vi "fpga_Fund Filter Constant.vi"() -> (0 "Total Delay":u8=24, 1 "Start":fxp<+/-,4,4>=1.0, 2 "LP2 delay":u8, 3 "LP1 delay":u8=2)   [LabVIEW 2012, in "NI_EP_Protection_FPGA.lvlib"]
uses:
  <vilib>/addons/Electrical Power/Protection/NI_EP_Protection_FPGA.lvlib
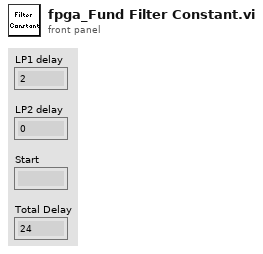
[diagram p1: front panel]
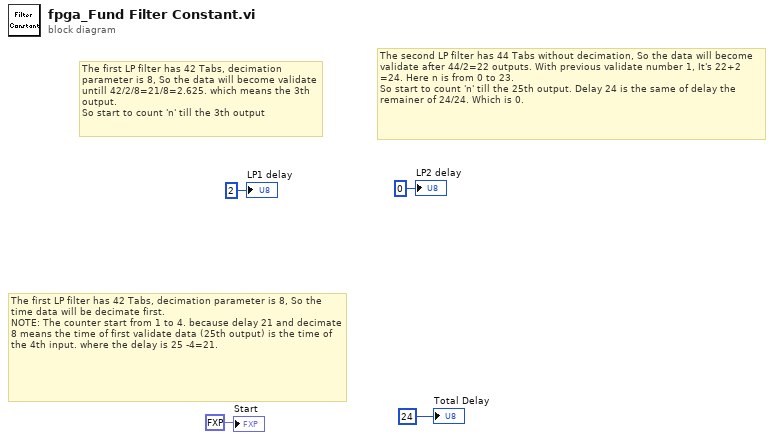
[diagram p0: block diagram]
diagram:
  # "The first LP filter has 42 Tabs, decimation parameter is 8, So the data will become validate untill 42/2/8=21/8=2.625. which means the 3th output.\nSo start to count 'n' till the 3th output"
  # "The second LP filter has 44 Tabs without decimation, So the data will become validate after 44/2=22 outputs. With previous validate number 1, It's 22+2 =24. Here n is from 0 to 23. \nSo start to count 'n' till the 25th output. Delay 24 is the same of delay the remainer of 24/24. Which is 0."
  # "The first LP filter has 42 Tabs, decimation parameter is 8, So the time data will be decimate first.\nNOTE: The counter start from 1 to 4. because delay 21 and decimate 8 means the time of first validate data (25th output) is the time of the 4th input. where the delay is 25 -4=21."
  "Start" <- fxp<+/-,4,4> 1.0 ("Start")
  "Total Delay" <- u8 24 ("Total Delay")
  "LP1 delay" <- u8 2 ("n-1[0..15]")
  "LP2 delay" <- u8 0 ("n-1[0..23]")
